vi "scale to range.vi"(4 "Max":dbl, 5 "High":dbl, 6 "Min":dbl, 7 "Low":dbl, 10 "In Signal":dbl) -> (2 "Output signal":dbl)   [LabVIEW 2017]
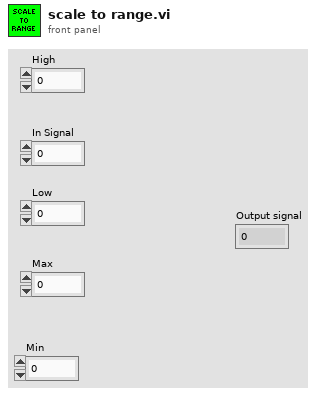
[diagram p1: front panel]
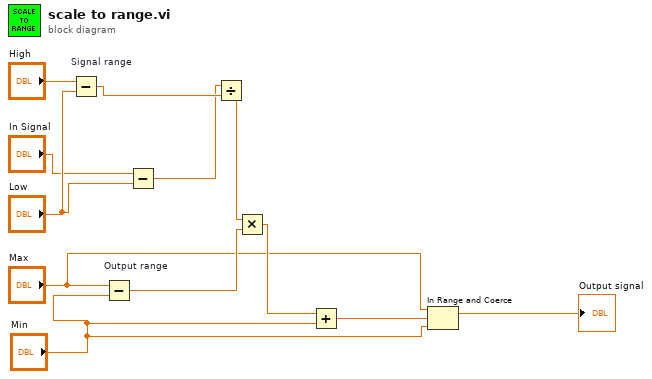
[diagram p0: block diagram]
diagram:
  n1 = Subtract "Signal range"(x="High", y="Low") -> (x-y=w9:dbl)
  n2 = Subtract "Output range"(x="Max", y="Min") -> (x-y=w7:dbl)
  n3 = Subtract(x="In Signal", y="Low") -> (x-y=w8:dbl)
  n4 = Divide(x=w8, y=w9) -> (x/y=w6:dbl)
  n5 = Multiply(x=w6, y=w7) -> (x*y=w5:dbl)
  n6 = Add(x=w5, y="Min") -> (x+y=w4:dbl)
  n7 = In Range and Coerce(upper limit="Max", x=w4, lower limit="Min") -> (coerced(x)=→"Output signal":dbl)  [unwired: 1 out]
